vi "Test Read Traces.vi"() -> ()   [LabVIEW 2013]
uses:
  <vilib>/lvdsc/historical/Read Traces (Numeric).vi
  <vilib>/lvdsc/NI_DSC.lvlib
panel:
  out "historical traces":T1(array[cluster]) {"data" format="%0.6f"; "timestamps" format="%<%X\n%x>T"}
  in  "options":T2={"interpolate data (F)"=TRUE, "extrapolate to now (F)"=FALSE, "remove data breaks (F)"=TRUE, "interpolation interval (1 s)"=1.0, "maintain trending info (T)"=FALSE} {"interpolation interval (1 s)" min=0.0 format="%0.2f"}
  in  "time interval":T3 {"stop timestamp (now)" format="%<%X\n%x>T"; "start timestamp" format="%<%X\n%x>T"}
  out "quality":i32[][](array[numeric])
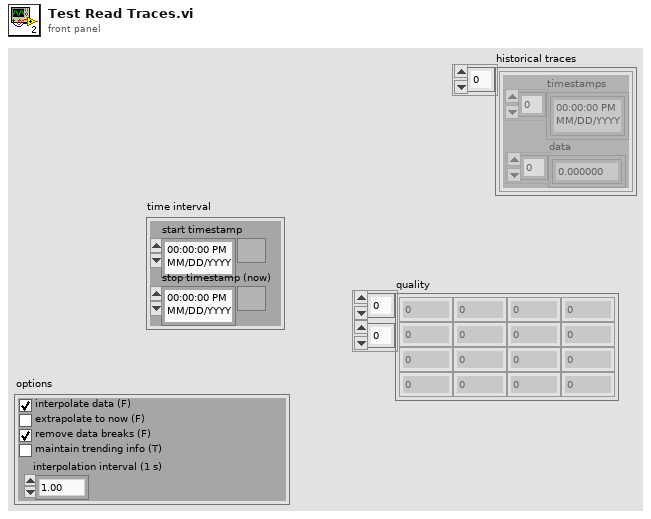
[diagram p1: front panel]
types:
  T1 = cluster{"timestamps":timestamp[], "data":dbl[]}[]
  T2 = cluster{"interpolate data (F)":bool, "extrapolate to now (F)":bool, "remove data breaks (F)":bool, "interpolation interval (1 s)":dbl, "maintain trending info (T)":bool}
  T3 = cluster{"start timestamp":timestamp, "stop timestamp (now)":timestamp}
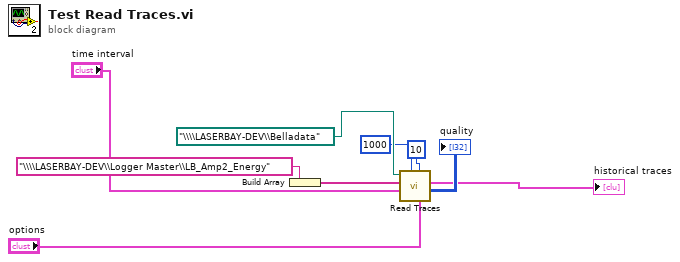
[diagram p0: block diagram]
diagram:
  n1 = Build Array("\\\\LASERBAY-DEV\\Logger Master\\LB_Amp2_Energy") -> (w2:string[])
  n2 = call-poly <vilib>:"Read Traces.vi"("options"="options", "timeout (30 s)"=10, "max points per trace (all)"=1000, "time interval"="time interval", "trace names"=w2, "database URL"=path "\\\\LASERBAY-DEV\\Belladata") -> ("quality"=→"quality":i32[][], "historical traces"=→"historical traces":T1)  [unwired: 2 in, 2 out]
